vi "SendEMail.vi"(8 "error in":errorcluster) -> (0 "error out":errorcluster)   [LabVIEW 2014]
uses:
  <vilib>/smtpClient/Set Message Text.vi
  <vilib>/smtpClient/LabVIEWSMTPClient.lvlib
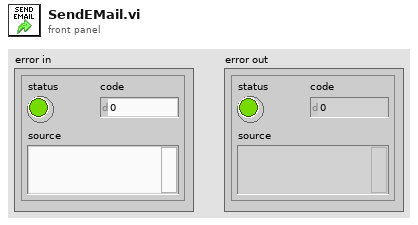
[diagram p1: front panel]
types:
  T1 = typedef "LabVIEWSMTPClient.lvlib/SmtpClientHandle.ctl" = refnum<k1>
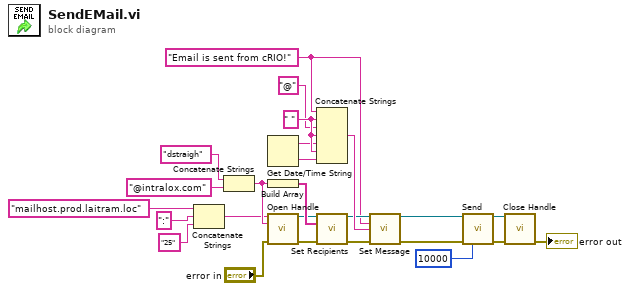
[diagram p0: block diagram]
diagram:
  w1 = "Email is sent from cRIO!" ("string")
  w24 = " "
  n1 = Concatenate Strings("mailhost.prod.laitram.loc" ("server address"), ":" ("string"), "25" ("from")) -> (w6:string)
  n2 = Concatenate Strings("dstraigh" ("string"), "@intralox.com" ("string")) -> (w20:string)
  n3 = Get Date/Time String() -> (date string=w23:string, time string=w25:string)  [unwired: 3 in]
  n4 = Build Array(w20) -> (w8:string[])
  n5 = call <vilib>:"Open Handle.vi"("server address"=w6, "from"=w20, "error in (no error)"="error in") -> ("handle out"=w7:T1, "error out"=w10:errorcluster)  [unwired: 11 in]
  n6 = Concatenate Strings(w1, w24, "@", w24, w23, w24, w25) -> (w21:string)
  n7 = call <vilib>:"Set Recipients.vi"("handle in"=w7, "to"=w8, "error in (no error)"=w10) -> ("handle out"=w9:T1, "error out"=w11:errorcluster)  [unwired: 11 in]
  n8 = call-poly <vilib>:"Set Message.vi"("handle in"=w9, "subject"=w1, "plain text message"=w21, "error in (no error)"=w11) -> ("handle out"=w12:T1, "error out"=w13:errorcluster)  [unwired: 10 in]
  n9 = call <vilib>:"Send.vi"("handle in"=w12, "error in (no error)"=w13, "timeout in ms (10000)"=10000) -> ("handle out"=w15:T1, "error out"=w16:errorcluster)  [unwired: 10 in, 1 out]
  n10 = call <vilib>:"Close Handle.vi"("handle in"=w15, "error in (no error)"=w16) -> ("error out"=→"error out":errorcluster)  [unwired: 12 in, 1 out]
